vi "RH_DCPower_ConfigureSequenceCapDC.vi"(7 "DCPower_SequenceParameters":T1 {"DeltaVoltage" format="%.6p"; "DeltaTime" format="%.6p"; "Voltage Stop" format="%.6p"; "Aperture_time" format="%.6p"; "Current_range" format="%.6p"; "Current" format="%.6p"; "Voltage_range" format="%.6p"; "Voltage Start" format="%.6p"}, 8 "error in (no error)":errorcluster, 9 "Peak duration (s)":dbl, 10 "channel name":string, 11 "DCPower Session In":refnum<k15>) -> (0 "error out":errorcluster, 1 "RecordLength":i32, 2 "num points":i32, 3 "DCPower Session Out":refnum<k15>)   [LabVIEW 2023, in "ResourceHandling.lvlib"]
uses:
  ResourceHandling.lvlib
  TypeDefs/RH_DCPower_SequenceParameters.ctl
  <instrlib>/niDCPower/nidcpower.llb/niDCPower Source Mode.ctl
  <instrlib>/niDCPower/nidcpower.llb/niDCPower Output Function.ctl
  <instrlib>/niDCPower/nidcpower.llb/niDCPower Aperture Time Units.ctl
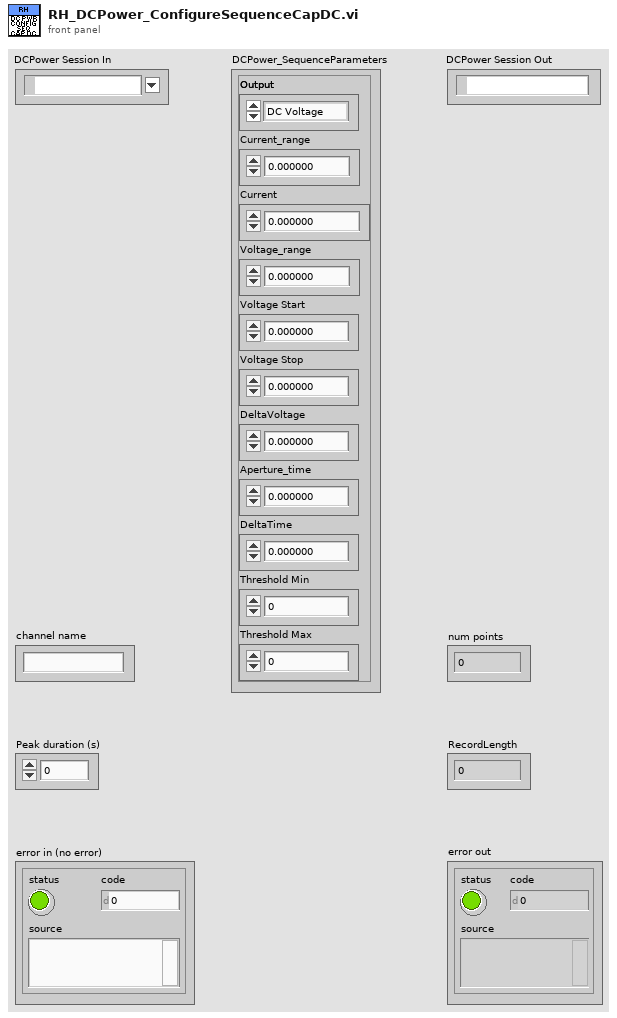
[diagram p1: front panel]
types:
  T1 = typedef "ResourceHandling.lvlib/RH_DCPower_SequenceParameters.ctl" = cluster{"Output":enum16{"DC Voltage", "DC Current"}, "Current_range":dbl, "Current":dbl, "Voltage_range":dbl, "Voltage Start":dbl, "Voltage Stop":dbl, "DeltaVoltage":dbl, "Aperture_time":dbl, "DeltaTime":dbl, "Threshold Min":dbl, "Threshold Max":dbl}
  T2 = typedef "niDCPower Aperture Time Units.ctl" = i32
  T3 = typedef "niDCPower Output Function.ctl" = i32
  T4 = typedef "niDCPower Source Mode.ctl" = i32
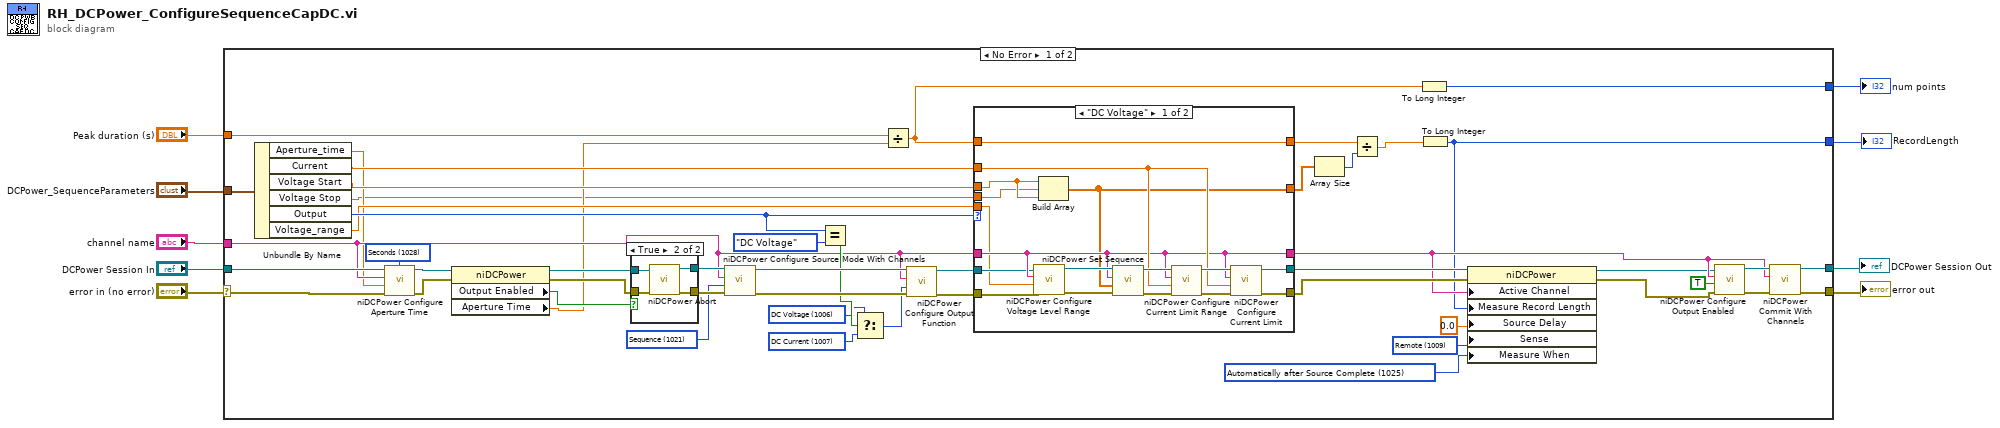
[diagram p0: block diagram]
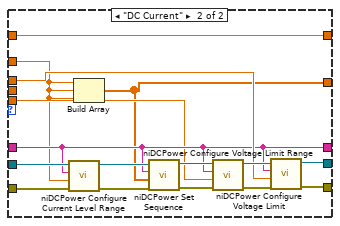
[diagram p2: hidden frame]
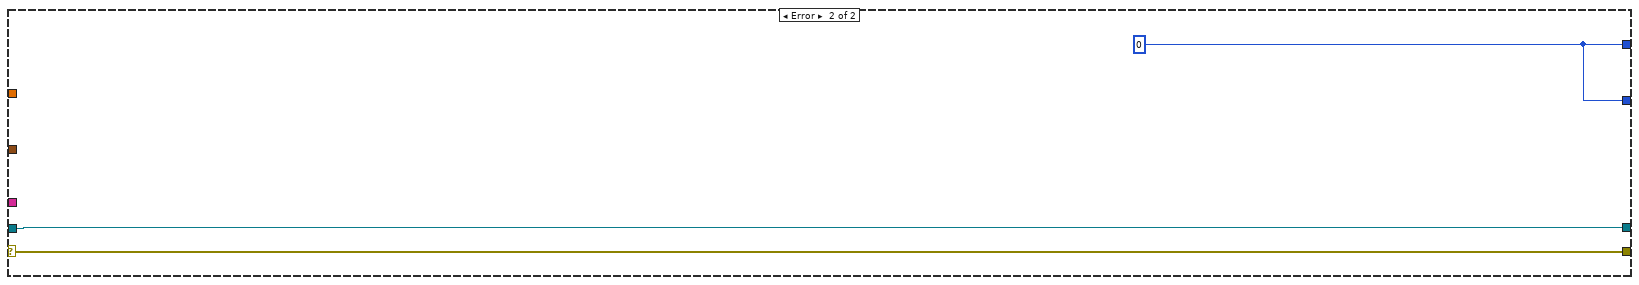
[diagram p4: hidden frame]
diagram:
  n1 = case shown="No Error" "error in (no error)" {
    selector: "error in (no error)" -> [w23 w101]
    tunnel: "DCPower Session In" -> [w22 w100]
    tunnel: "channel name" -> [w21 _]
    tunnel: "DCPower_SequenceParameters" -> [w47 _]
    tunnel: "Peak duration (s)" -> [w48 _]
    tunnel: [w34 w99] -> w5
    tunnel: [w33 w101] -> w4
    tunnel: [w32 w100] -> w1
    tunnel: [w25 w99] -> w3
    frame No Error {
      w10 = 1025 items=["Automatically after Source Complete"=1025, "On Demand"=1026, "On Measure Trigger"=1027] ("Measurement:Advanced:Measure When")
      w24 = T2 1028 items=["Seconds"=1028, "Powerline Cycles"=1029] ("aperture time units")
      w36 = 1009 items=["Local"=1008, "Remote"=1009] ("Measurement:Sense")
      w40 = T3 1007 items=["DC Voltage"=1006, "DC Current"=1007, "Pulse Voltage"=1049, "Pulse Current"=1050] ("output function")
      w39 = T3 1006 items=["DC Voltage"=1006, "DC Current"=1007, "Pulse Voltage"=1049, "Pulse Current"=1050] ("output function")
      w44 = T4 1021 items=["Single Point"=1020, "Sequence"=1021] ("source mode")
      n2 = Unbundle By Name(w47) -> ("Aperture_time"=w20:dbl, "Current"=w46:dbl, "Voltage Start"=w45:dbl, "Voltage Stop"=w11:dbl, "Output"=w43:enum16{"DC Voltage", "DC Current"}, "Voltage_range"=w30:dbl)
      n3 = call <instrlib>:"niDCPower Configure Aperture Time.vi"("aperture time units"=w24, "error in (no error)"=w23, "aperture time"=w20, "channel name"=w21, "instrument handle"=w22) -> ("error out"=w19:errorcluster, "instrument handle out"=w18:refnum<k15>)  [unwired: 5 in]
      n4 = property class="niDCPower"(reference=w18, error in=w19) -> (reference out=w16:refnum<k15>, error out=w15:errorcluster, "Output Enabled"=w17:bool, "Aperture Time"=w14:dbl)
      n5 = case shown="True" w17 {
        tunnel: [w93 w98] -> w50
        tunnel: [w94 w97] -> w49
        tunnel: w16 -> [w94 w96]
        tunnel: w15 -> [w93 w95]
        frame False {
        }
        frame True {
          n6 = call <instrlib>:"niDCPower Abort.vi"("error in (no error)"=w95, "instrument handle"=w96) -> ("error out"=w98:errorcluster, "instrument handle out"=w97:refnum<k15>)  [unwired: 8 in]
        }
      }
      n7 = call <instrlib>:"niDCPower Configure Source Mode With Channels.vi"("error in (no error)"=w50, "source mode"=w44, "channel name"=w21, "instrument handle"=w49) -> ("error out"=w53:errorcluster, "instrument handle out"=w54:refnum<k15>)  [unwired: 6 in]
      n8 = Equal?(x=w43, y=enum16{"DC Voltage", "DC Current"}."DC Voltage") -> (x = y?=w41:bool)
      n9 = Select(t=w39, s=w41, f=w40) -> (s? t:f=w38:T3)
      n10 = Divide(x=w48, y=w14) -> (x/y=w35:dbl)
      n11 = call <instrlib>:"niDCPower Configure Output Function.vi"("error in (no error)"=w53, "output function"=w38, "channel name"=w21, "instrument handle"=w54) -> ("error out"=w52:errorcluster, "instrument handle out"=w51:refnum<k15>)  [unwired: 6 out]
      n12 = case shown="\"DC Voltage\"" w43 {
        tunnel: w21 -> [w67 w80]
        tunnel: w45 -> [w62 w81]
        tunnel: w46 -> [w70 w78]
        tunnel: [w69 w83] -> w59
        tunnel: [w68 w85] -> w58
        tunnel: [w67 w80] -> w31
        tunnel: w35 -> [w66 w92]
        tunnel: [w66 w92] -> w29
        tunnel: w52 -> [w65 w91]
        tunnel: w51 -> [w64 w90]
        tunnel: w11 -> [w61 _]
        tunnel: w30 -> [w63 w79]
        tunnel: [w60 w77] -> w27
        frame "DC Voltage" {
          n13 = call <instrlib>:"niDCPower Configure Voltage Level Range.vi"("error in (no error)"=w65, "voltage level range"=w63, "channel name"=w67, "instrument handle"=w64) -> ("error out"=w72:errorcluster, "instrument handle out"=w71:refnum<k15>)  [unwired: 6 in]
          n14 = Build Array(w62, w61, w62) -> (w60:dbl[])
          n15 = call <instrlib>:"niDCPower Set Sequence.vi"("error in (no error)"=w72, "values"=w60, "channel name"=w67, "instrument handle"=w71) -> ("error out"=w76:errorcluster, "instrument handle out"=w74:refnum<k15>)  [unwired: 1 in, 5 out]
          n16 = call <instrlib>:"niDCPower Configure Current Limit Range.vi"("error in (no error)"=w76, "current limit range"=w70, "channel name"=w67, "instrument handle"=w74) -> ("error out"=w75:errorcluster, "instrument handle out"=w73:refnum<k15>)  [unwired: 6 in]
          n17 = call <instrlib>:"niDCPower Configure Current Limit.vi"("error in (no error)"=w75, "current limit"=w70, "channel name"=w67, "instrument handle"=w73) -> ("error out"=w68:errorcluster, "instrument handle out"=w69:refnum<k15>)  [unwired: 1 in, 5 out]
        }
        frame "DC Current" {
          n18 = call <instrlib>:"niDCPower Configure Current Level Range.vi"("error in (no error)"=w91, "current level range"=w78, "channel name"=w80, "instrument handle"=w90) -> ("error out"=w89:errorcluster, "instrument handle out"=w88:refnum<k15>)  [unwired: 6 in]
          n19 = Build Array(w78, w78, w78) -> (w77:dbl[])
          n20 = call <instrlib>:"niDCPower Set Sequence.vi"("error in (no error)"=w89, "values"=w77, "channel name"=w80, "instrument handle"=w88) -> ("error out"=w86:errorcluster, "instrument handle out"=w87:refnum<k15>)  [unwired: 1 in, 5 out]
          n21 = call <instrlib>:"niDCPower Configure Voltage Limit Range.vi"("error in (no error)"=w86, "voltage limit range"=w79, "channel name"=w80, "instrument handle"=w87) -> ("error out"=w82:errorcluster, "instrument handle out"=w84:refnum<k15>)  [unwired: 6 in]
          n22 = call <instrlib>:"niDCPower Configure Voltage Limit.vi"("error in (no error)"=w82, "voltage limit"=w81, "channel name"=w80, "instrument handle"=w84) -> ("error out"=w85:errorcluster, "instrument handle out"=w83:refnum<k15>)  [unwired: 6 in]
        }
      }
      n23 = Array Size(array=w27) -> (size(s)=w26:i32)
      n24 = Divide(x=w29, y=w26) -> (x/y=w28:dbl)
      n25 = To Long Integer(number=w35) -> (32bit integer=w34:i32)
      n26 = To Long Integer(number=w28) -> (32bit integer=w25:i32)
      n27 = property class="niDCPower"(reference=w59, error in=w58, "Active Channel"=w31, "Measure Record Length"=w25, "Source Delay"=0.0 ("Source:Advanced:Source Delay"), "Sense"=w36, "Measure When"=w10) -> (reference out=w13:refnum<k15>, error out=w12:errorcluster)
      n28 = call <instrlib>:"niDCPower Configure Output Enabled.vi"("error in (no error)"=w12, "output enabled"=TRUE, "channel name"=w31, "instrument handle"=w13) -> ("error out"=w57:errorcluster, "instrument handle out"=w56:refnum<k15>)  [unwired: 6 in]
      n29 = call <instrlib>:"niDCPower Commit With Channels.vi"("error in (no error)"=w57, "channel name"=w31, "instrument handle"=w56) -> ("error out"=w33:errorcluster, "instrument handle out"=w32:refnum<k15>)  [unwired: 7 in]
    }
    frame Error {
      w99 = 0
    }
  }
  "error out" <- w4
  "num points" <- w5
  "RecordLength" <- w3
  "DCPower Session Out" <- w1
